vi "Arm_Control.vi"() -> ()   [LabVIEW 2012]
uses:
  StateMachineEnum.ctl
  Robot Global Data.vi
panel:
  in  "ArmBackSpeed":dbl=-0.32
  in  "ArmForwardSpeed":dbl=0.32
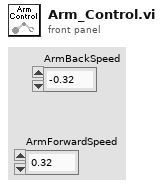
[diagram p1: front panel]
types:
  T1 = typedef "StateMachineEnum.ctl" = enum16{"Init", "Idle", "Start", "Do", "Stop"}
  T2 = typedef "WPI_MotorControlDeviceRef.ctl" = cluster{"DeviceStatus":errorcluster, "Type":enum16{"PWM", "CAN"}, "PWM":cluster{"Digital Module":T3, "PWM Channel":T4, "DeadBand":T5}, "CAN":cluster{"Device Number":u8, "Control Mode":T6, "Semaphore":T7, "Max Vout":dbl}, "Invert":bool, "TransformRef":T8, "InvTransformRef":T8}
  T3 = typedef "FPGA_TypedefDigitalModule.ctl" = enum16{"Digital Module 1", "Digital Module 2"}
  T4 = typedef "FPGA_DIOPWMChannel.ctl" = enum8{"PWM 1", "PWM 2", "PWM 3", "PWM 4", "PWM 5", "PWM 6", "PWM 7", "PWM 8", "PWM 9", "PWM 10", "Invalid"}
  T5 = typedef "WPI_PWMDeadband.ctl" = cluster{"Name":string, "maxPositivePwm":i32, "minPositivePwm":i32, "centerPwm":i32, "maxNegativePwm":i32, "minNegativePwm":i32, "angularRange":u16}
  T6 = typedef "WPI_CANJaguar_ControlMode.ctl" = enum8{"Percent VBus", "Current", "Speed", "Position", "Voltage"}
  T7 = typedef "Semaphore RefNum" = refnum<k1>
  T8 = typedef "WPI_PWMTransform_ConPane.ctl" = refnum<vi>
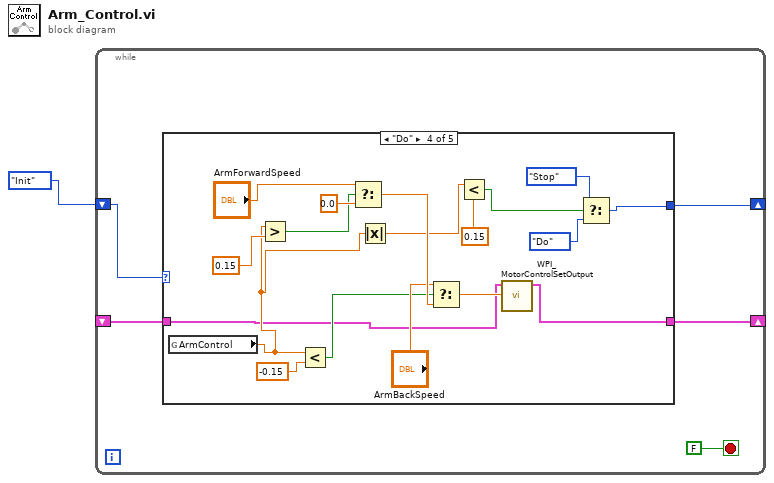
[diagram p0: block diagram]
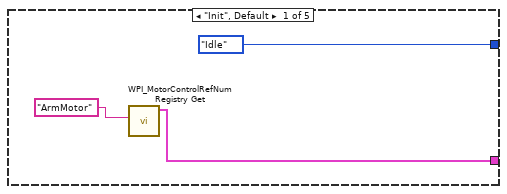
[diagram p2: hidden frame]
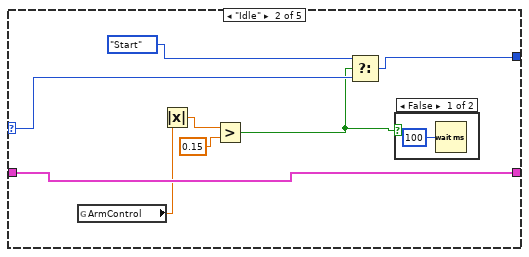
[diagram p3: hidden frame]
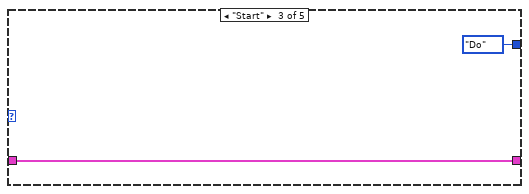
[diagram p5: hidden frame]
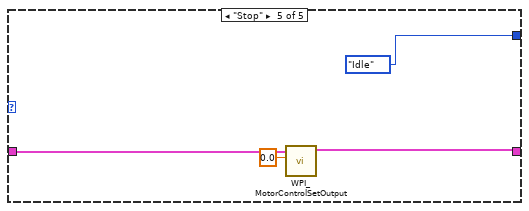
[diagram p6: hidden frame]
diagram:
  n1 = while {
    shift-right: [w5] -> _
    shift-left: _ -> [w2]
    shift-right: [w4] -> _
    shift-left: StateMachineEnum."Init" ("State") -> [w3]
    stop <- FALSE stop-if-true
    n2 = case shown="\"Do\"" w3 {
      selector: w3 -> [_ w16 _ _ _]
      tunnel: [w8 w14 w20 w21 w40] -> w5
      tunnel: [StateMachineEnum."Idle" ("State") w15 StateMachineEnum."Do" ("State") w33 StateMachineEnum."Idle" ("State")] -> w4
      tunnel: w2 -> [_ w14 w20 w22 w41]
      frame "Init", Default {
        n3 = call <vilib>:"WPI_MotorControlRefNum Registry Get.vi"("refnum name"="ArmMotor") -> ("MotorControlDevRef"=w8:T2)  [unwired: 9 in, 1 out]
      }
      frame "Idle" {
        n4 = global read "Robot Global Data.vi" "ArmControl"() -> (w10:dbl)
        n5 = Absolute Value(x=w10) -> (abs(x)=w13:dbl)
        n6 = Greater?(x=w13, y=0.15) -> (0:w11:bool)
        n7 = Select(t=StateMachineEnum."Start" ("State"), s=w11, f=w16) -> (s? t:f=w15:T1)
        n8 = case shown="False" w11 {
          frame False {
            n9 = Wait (ms)(milliseconds to wait=u32 100) -> ()  [unwired: 1 out]
          }
          frame True {
          }
        }
      }
      frame "Start" {
      }
      frame "Do" {
        n10 = global read "Robot Global Data.vi" "ArmControl"() -> (w23:dbl)
        n11 = Greater?(x=w23, y=0.15) -> (0:w29:bool)
        n12 = Less?(x=w23, y=-0.15) -> (x < y?=w27:bool)
        n13 = Select(t="ArmForwardSpeed", s=w29, f=0.0) -> (s? t:f=w32:dbl)
        n14 = Absolute Value(x=w23) -> (abs(x)=w26:dbl)
        n15 = Select(t="ArmBackSpeed", s=w27, f=w32) -> (s? t:f=w36:dbl)
        n16 = Less?(x=w26, y=0.15) -> (x < y?=w24:bool)
        n17 = call <vilib>:"WPI_MotorControlSetOutput.vi"("Output"=w36, "MotorControlDevRef"=w22) -> ("MotorControlDevRef"=w21:T2)  [unwired: 7 in, 2 out]
        n18 = Select(t=StateMachineEnum."Stop" ("State"), s=w24, f=StateMachineEnum."Do" ("State")) -> (s? t:f=w33:T1)
      }
      frame "Stop" {
        n19 = call <vilib>:"WPI_MotorControlSetOutput.vi"("Output"=0.0, "MotorControlDevRef"=w41) -> ("MotorControlDevRef"=w40:T2)  [unwired: 7 in, 2 out]
      }
    }
  }
